vi "ROI thickener.vi"(2 "error in":errorcluster caption="Fehler (Ausgang)", 3 "ROI Descriptor in":T2) -> (0 "error out":errorcluster, 1 "ROI Descriptor out":T1 {"Contours"."Type" items=["No Selection", "Point", "Line", "Rectangle", "Oval", "Polygon", "Freehand Region", "Annulus", "Unused2", "Unused3", "Broken Line", "Freehand Line", "Rotated Rectangle"]})   [LabVIEW 2013]
uses:
  <vilib>/vision/NI_Vision_Development_Module.lvlib
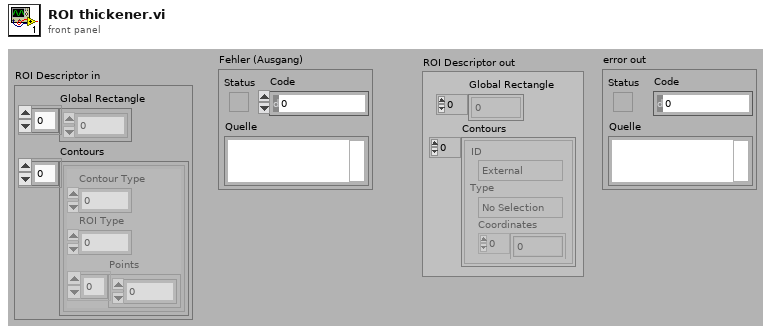
[diagram p1: front panel]
types:
  T1 = typedef "ROI Descriptor" = cluster{"Global Rectangle":i32[], "Contours":cluster{"ID":enum32{"External", "Internal"}, "Type":u32, "Coordinates":i32[]}[]}
  T2 = cluster{"Global Rectangle":i32[], "Contours":cluster{"Contour Type":u32, "ROI Type":u32, "Points":i32[]}[]}
  T3 = cluster{"Origin":cluster{"X":sgl, "Y":sgl}, "Angle (deg)":sgl, "Axis Reference":u32}
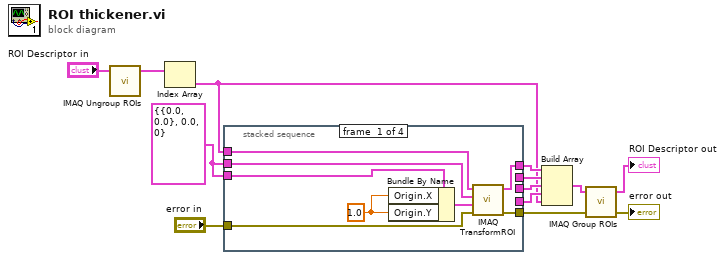
[diagram p0: block diagram]
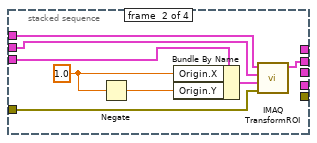
[diagram p2: hidden frame]
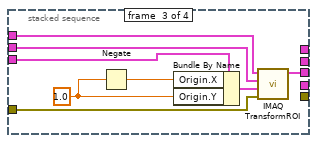
[diagram p3: hidden frame]
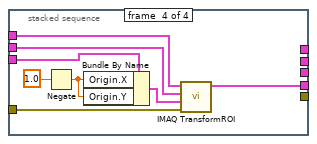
[diagram p4: hidden frame]
diagram:
  w13 = T3 {"Origin"={"X"=0.0, "Y"=0.0}, "Angle (deg)"=0.0, "Axis Reference"=0} ("Base Reference")
  n1 = call "IMAQ Ungroup ROIs"("ROI Descriptor"="ROI Descriptor in") -> ("ROI Descriptors out"=w2:T1[])  [unwired: 3 in, 1 out]
  n2 = Index Array(array=w2) -> (element=w1:T1)  [unwired: 1 in]
  n3 = stacked-sequence {
    tunnel: "error in" -> [w21 w29 w37 w45]
    tunnel: w13 -> [w20 w27 w36 w44]
    tunnel: w1 -> [w14 w26 w35 w43]
    tunnel: [w19 _ _ _] -> w4
    tunnel: [_ w25 _ _] -> w5
    tunnel: [_ _ w33 _] -> w6
    tunnel: [_ _ _ w41] -> w7
    tunnel: [w18 _ _ _] -> w11
    tunnel: w13 -> [w17 w23 w31 w39]
    frame #0 {
      w15 = sgl 1.0 ("Origin.X")
      n4 = Bundle By Name(cluster=w17, "Origin.X"=w15, "Origin.Y"=w15) -> (w16:T3)
      n5 = call "IMAQ TransformROI"("error in (no error)"=w21, "New Reference"=w16, "Base Reference"=w20, "ROI Descriptor"=w14) -> ("error out"=w18:errorcluster, "ROI Descriptor out"=w19:T1)  [unwired: 6 in]
    }
    frame #1 {
      w24 = 1.0 ("X")
      n6 = Negate(x=w24) -> (-x=w28:dbl)
      n7 = Bundle By Name(cluster=w23, "Origin.X"=w24, "Origin.Y"=w28) -> (w22:T3)
      n8 = call "IMAQ TransformROI"("error in (no error)"=w29, "New Reference"=w22, "Base Reference"=w27, "ROI Descriptor"=w26) -> ("ROI Descriptor out"=w25:T1)  [unwired: 6 in, 1 out]
    }
    frame #2 {
      w32 = 1.0 ("x")
      n9 = Negate(x=w32) -> (-x=w34:dbl)
      n10 = Bundle By Name(cluster=w31, "Origin.X"=w34, "Origin.Y"=w32) -> (w30:T3)
      n11 = call "IMAQ TransformROI"("error in (no error)"=w37, "New Reference"=w30, "Base Reference"=w36, "ROI Descriptor"=w35) -> ("ROI Descriptor out"=w33:T1)  [unwired: 6 in, 1 out]
    }
    frame #3 {
      n12 = Negate(x=1.0) -> (-x=w42:dbl)
      n13 = Bundle By Name(cluster=w39, "Origin.X"=w42, "Origin.Y"=w42) -> (w38:T3)
      n14 = call "IMAQ TransformROI"("error in (no error)"=w45, "New Reference"=w38, "Base Reference"=w44, "ROI Descriptor"=w43) -> ("ROI Descriptor out"=w41:T1)  [unwired: 6 in, 1 out]
    }
  }
  n15 = Build Array(w4, w5, w6, w7, w1) -> (w9:T1[])
  n16 = call "IMAQ Group ROIs"("error in (no error)"=w11, "ROI Descriptors"=w9) -> ("error out"=→"error out":errorcluster, "ROI Descriptor out"=→"ROI Descriptor out":T1)  [unwired: 2 in]
